vi "Mascara_Serial.vi"(7 "error in":errorcluster, 9 "Serial":string) -> (0 "error out":errorcluster, 1 "Offset":i32, 2 "Mask_Ok?":bool)   [LabVIEW 2021]
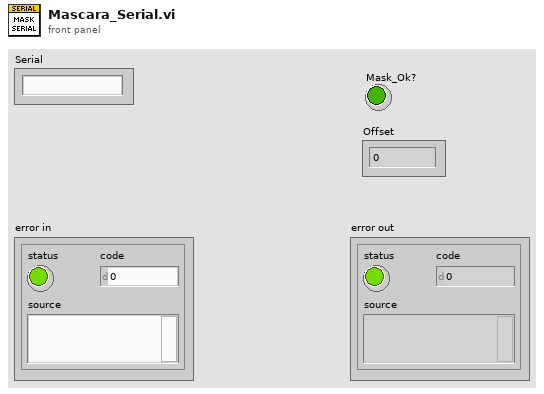
[diagram p1: front panel]
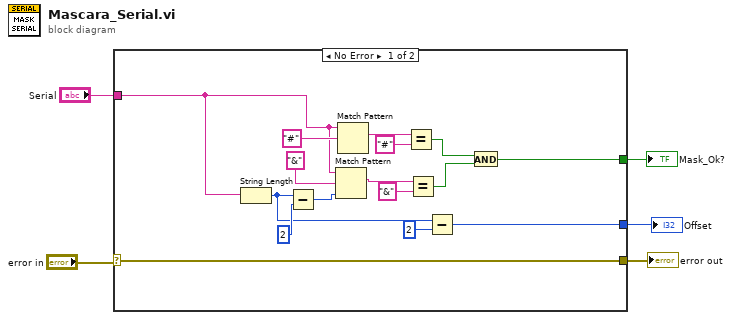
[diagram p0: block diagram]
diagram:
  n1 = case shown="No Error" "error in" {
    selector: "error in" -> [w12 w22]
    tunnel: [w12 w22] -> w4
    tunnel: [w8 _] -> w3
    tunnel: [w7 _] -> w2
    tunnel: "Serial" -> [w6 _]
    frame No Error {
      n2 = String Length(string=w6) -> (length=w9:i32)
      n3 = Subtract(x=w9, y=2) -> (x-y=w11:i32)
      n4 = Match Pattern(string=w6, regular expression="&", offset (0)=w11) -> (match substring=w16:string)  [unwired: 3 out]
      n5 = Match Pattern(string=w6, regular expression="#") -> (match substring=w19:string)  [unwired: 1 in, 3 out]
      n6 = Equal?(x=w19, y="#") -> (x = y?=w15:bool)
      n7 = Equal?(x=w16, y="&") -> (x = y?=w14:bool)
      n8 = Subtract(x=w9, y=2) -> (x-y=w7:i32)
      n9 = And(x=w15, y=w14) -> (x .and. y?=w8:bool)
    }
    frame Error {
    }
  }
  "error out" <- w4
  "Mask_Ok?" <- w3
  "Offset" <- w2
